vi "Set Revision From Module Information.vi"(8 "error in":errorcluster, 10 "module information":T1, 11 "routing and faulting in":T3 format="%.0x") -> (0 "error out":errorcluster, 3 "routing and faulting out":T3 format="%.0x")   [LabVIEW 2020, in "Routing and Faulting Scripting.lvlib"]
uses:
  Routing and Faulting Scripting.lvlib
  <vilib>/NI VeriStand/Custom Device API/Custom Device Item Ref.ctl
  Types/Module Information.ctl
  Shared/Routing and Faulting Hardware API/Types/Possible Connections for Endpoint.ctl
  <vilib>/NI VeriStand/Custom Device API/Custom Device API.lvlib
  Shared/Routing and Faulting Hardware API/Routing and Faulting Hardware API.lvlib
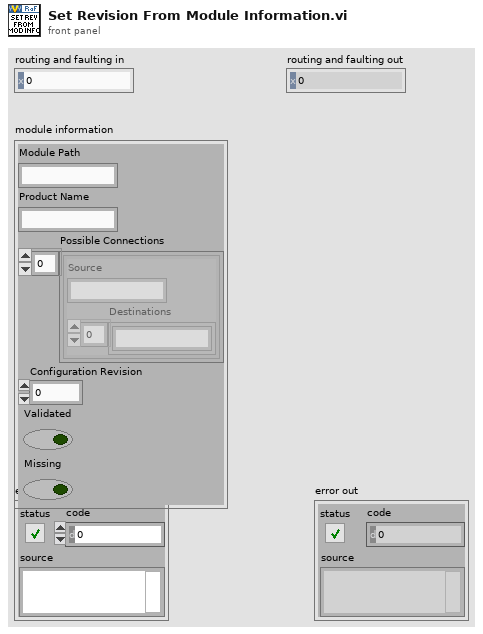
[diagram p1: front panel]
types:
  T1 = typedef "Routing and Faulting Scripting.lvlib/Module Information.ctl" = cluster{"Module Path":string, "Product Name":string, "Possible Connections":T2[], "Configuration Revision":u32, "Validated":bool, "Missing":bool}
  T2 = typedef "Routing and Faulting Hardware API.lvlib/Possible Connections for Endpoint.ctl" = cluster{"Source":string, "Destinations":string[]}
  T3 = typedef "Custom Device API.lvlib/Custom Device Item Ref.ctl" = u64
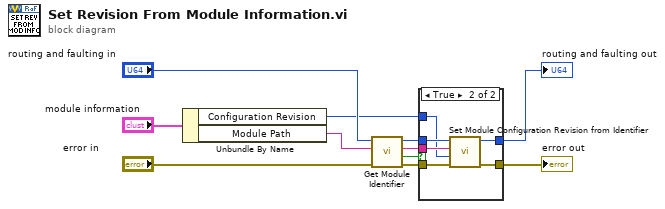
[diagram p0: block diagram]
diagram:
  n1 = Unbundle By Name("module information") -> ("Configuration Revision"=w4:u32, "Module Path"=w10:string)
  n2 = call "Get Module Identifier.vi"("error in"="error in", "module path"=w10, "routing and faulting in"="routing and faulting in") -> ("error out"=w7:errorcluster, "found?"=w1:bool, "module identifier"=w5:string, "routing and faulting out"=w6:T3)  [unwired: 5 in]
  n3 = case shown="True" w1 {
    tunnel: w7 -> [w12 w19]
    tunnel: w6 -> [w13 w18]
    tunnel: w5 -> [_ w17]
    tunnel: w4 -> [_ w16]
    tunnel: [w12 w15] -> w3
    tunnel: [w13 w14] -> w2
    frame False {
    }
    frame True {
      n4 = call "Set Module Configuration Revision from Identifier.vi"("error in"=w19, "revision"=w16, "module identifier"=w17, "routing and faulting in"=w18) -> ("error out"=w15:errorcluster, "routing and faulting out"=w14:T3)  [unwired: 6 in]
    }
  }
  "routing and faulting out" <- w2
  "error out" <- w3
